vi "Create Output File Names (SubVI).vi"(11 "File Name Prefix":T1={"DateTimeStamp"="DateTimeStamp", "Genotype 1"="genotype1", "Genotype 2"="genotype2", "Rig Name"="stimulationMode", "STIM Mode"="t21", "Light Intensity (%)"=100, "Pixel Resolution (um/pixel)"=100.0, "Gamma"=0.2, "Yoked File Name"="none", "Yoked File Enable"=FALSE, "Output Folder Name"=path "", "Frame Number"=0, "Time Stamp (us)"=0, "Exp STOP"=0, "Contour"=[], "SPINE"=[], "Larvae ID"=[], "Larvae Valid?"=[], "Image Height"=0, "Image Width"=0, "Pixel Intensity Low"=0, "Pixel Intensity High"=0, "Box Side Low"=0, "Box Side High"=0, "Box W+L Low"=0, "Box W+L High"=0, "Area Low"=0, "Area High"=0, "N SPINE"=0, "BG SUB TH"=0, "Min Contour Points"=0, "XM1"=0.0, "YM1"=0.0, "XM2"=0.0, "YM2"=0.0, "XOFF"=0.0, "YOFF"=0.0}) -> (0 "SPINE File REF":refnum<file>, 1 "Movie File Path":path, 3 "Contour File REF":refnum<file>)   [LabVIEW 2015]
uses:
  Controls (HOST)/File Name Prefix.ctl
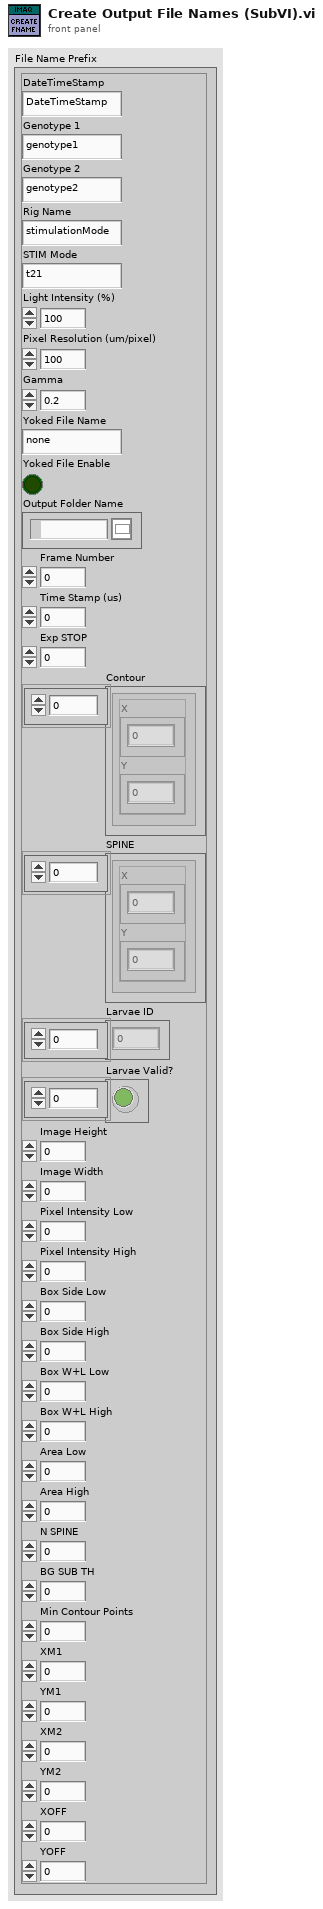
[diagram p1: front panel]
types:
  T1 = typedef "File Name Prefix.ctl" = cluster{"DateTimeStamp":string, "Genotype 1":string, "Genotype 2":string, "Rig Name":string, "STIM Mode":string, "Light Intensity (%)":i32, "Pixel Resolution (um/pixel)":dbl, "Gamma":dbl, "Yoked File Name":string, "Yoked File Enable":bool, "Output Folder Name":path, "Frame Number":u64, "Time Stamp (us)":u64, "Exp STOP":i32, "Contour":cluster{"X":i32[], "Y":i32[]}[], "SPINE":cluster{"X":dbl[], "Y":dbl[]}[], "Larvae ID":u32[], "Larvae Valid?":bool[], "Image Height":i32, "Image Width":i32, "Pixel Intensity Low":i32, "Pixel Intensity High":i32, "Box Side Low":i32, "Box Side High":i32, "Box W+L Low":i32, "Box W+L High":i32, "Area Low":i32, "Area High":i32, "N SPINE":i32, "BG SUB TH":i32, "Min Contour Points":i32, "XM1":dbl, "YM1":dbl, "XM2":dbl, "YM2":dbl, "XOFF":dbl, "YOFF":dbl}
  T2 = enum16{"open", "replace", "create", "open or create", "replace or create", "replace or create with confirmation"}
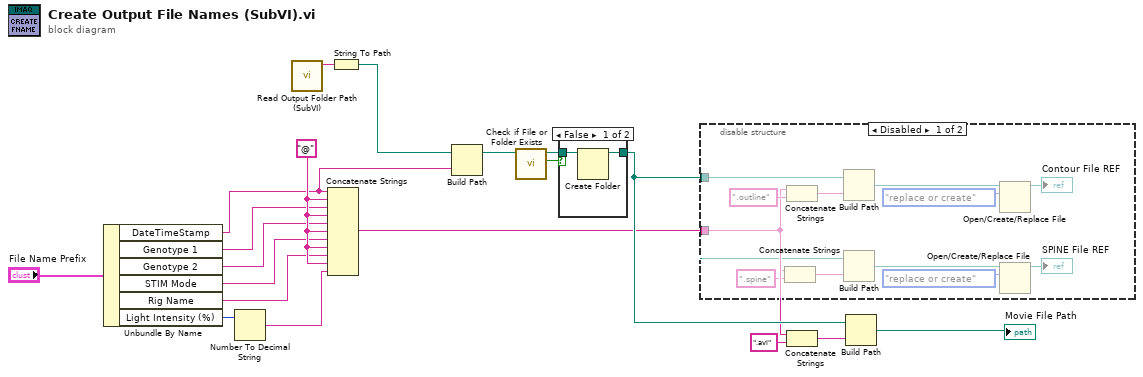
[diagram p0: block diagram]
diagram:
  w12 = "@" ("string")
  n1 = Unbundle By Name("File Name Prefix") -> ("DateTimeStamp"=w3:string, "Genotype 1"=w10:string, "Genotype 2"=w9:string, "STIM Mode"=w6:string, "Rig Name"=w7:string, "Light Intensity (%)"=w8:i32)
  n2 = Number To Decimal String(number=w8) -> (decimal integer string=w5:string)  [unwired: 1 in]
  n3 = call "Read Output Folder Path (SubVI).vi"() -> ("Output Folder"=w2:string)  [unwired: 11 in]
  n4 = Concatenate Strings(w3, w12, w10, w12, w9, w12, w6, w12, w7, w12, w5) -> (w13:string)
  n5 = String To Path(string=w2) -> (path=w1:path)
  n6 = Build Path(base path=w1, name or relative path=w3) -> (appended path=w4:path)
  n7 = call <vilib>:"Check if File or Folder Exists.vi"("path"=w4) -> ("file or folder exists?"=w19:bool, "dup path"=w18:path)  [unwired: 8 in, 1 out]
  n8 = case shown="False" w19 {
    tunnel: w18 -> [w21 w22]
    tunnel: [w20 w22] -> w15
    frame False {
      n9 = Create Folder(path (use dialog)=w21) -> (created path=w20:path)  [unwired: 2 in, 2 out]
    }
    frame True {
    }
  }
  n10 = disable-structure shown="Disabled" {
    disable-tunnel: w15 -> [w24 _]
    disable-tunnel: w13 -> [w23 _]
    frame Disabled {
      n11 = Concatenate Strings(w23, ".spine" ("string")) -> (w27:string)
      n12 = Concatenate Strings(w23, ".outline" ("string")) -> (w25:string)
      n13 = Build Path(base path=w24, name or relative path=w25) -> (appended path=w29:path)
      n14 = Build Path(base path=w24, name or relative path=w27) -> (appended path=w30:path)
      n15 = Open/Create/Replace File(file path (use dialog)=w29, operation (0:open)=T2."replace or create") -> (refnum out=→"Contour File REF":refnum<file>)  [unwired: 4 in, 2 out]
      n16 = Open/Create/Replace File(file path (use dialog)=w30, operation (0:open)=T2."replace or create") -> (refnum out=→"SPINE File REF":refnum<file>)  [unwired: 4 in, 2 out]
    }
    frame Enabled {
    }
  }
  n17 = Concatenate Strings(w13, ".avi" ("string")) -> (w17:string)
  n18 = Build Path(base path=w15, name or relative path=w17) -> (appended path=→"Movie File Path":path)
